vi "XYZ Software.vi"() -> ()   [LabVIEW 2020]
doc: "This was the initial version checking out system parameters and figuring out what each ASCII command does. The other file within this folder is setup to be able to send consecutive commands to the scanning rig controller."
uses:
  <instrlib>/Arcus Ethernet Driver 1.0.0/ArcusEthernetComm/classes/Controller/_Controller.lvclass
panel:
  in  "Program Stop":bool
  in  "Tab Control":T1(tab)
  in  "Scanning Rig Connection":T2
  out "Scanning Rig Disconnection":T2
  out "Current Z Vel (pps)":string
  out "Current Y Vel (pps)":string
  out "Current X Vel (pps)":string
  in  "Set HS Vel (pps)":string
  out "Current Decel (ms^2)":string
  out "Current LS Vel (pps)":string
  out "Current HS Vel (pps)":string
  in  "Set Accel (ms^2)":string
  out "Current Accel (ms^2)":string
  out "Home":bool
  out "Current Z Position":string
  out "Current X Position":string
  out "Current Y Position":string
  in  "Safe Motion Stop":bool
  in  "Direction":string(combo)
  in  "Axis":enum16{"X", "Y", "Z"}(ring)
  in  "Move":bool
  in  "Number of Z Steps":string
  in  "Number of Y Steps":string
  in  "Number of X Steps":string
  out "Z":bool
  out "Y":bool
  out "X":bool
  in  "Home":bool
  in  "Axis":enum16{"X", "Y", "Z"}(ring)
  in  "Direction":string(combo)
  # "`"
  # "GREEN - Operational\nRED - Activate Safe Stop"
  # "HOMING FUNCTION HAS MULTIPLE MODES\nSEE MANUAL"
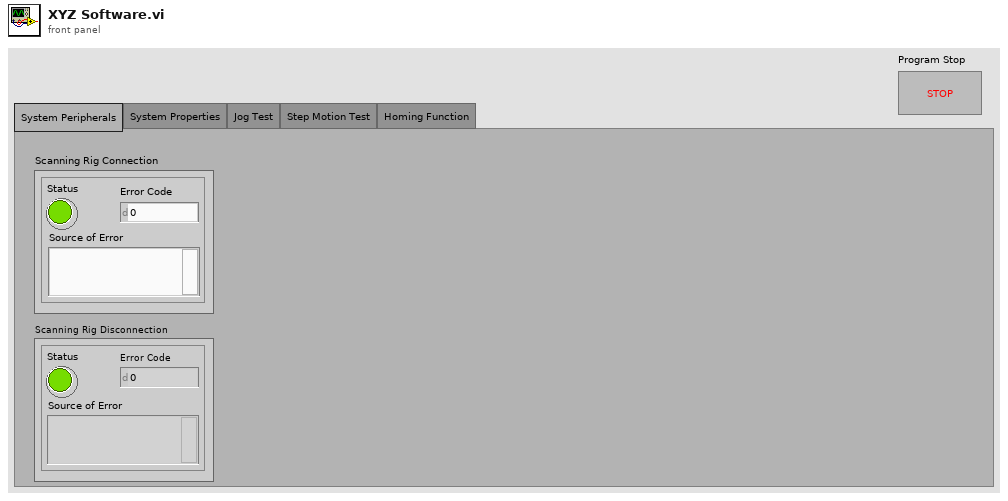
[diagram p1: front panel]
types:
  T1 = enum32{"System Peripherals", "System Properties", "Jog Test", "Step Motion Test", "Homing Function"}
  T2 = cluster{"Status":bool, "Error Code":i32, "Source of Error":string}
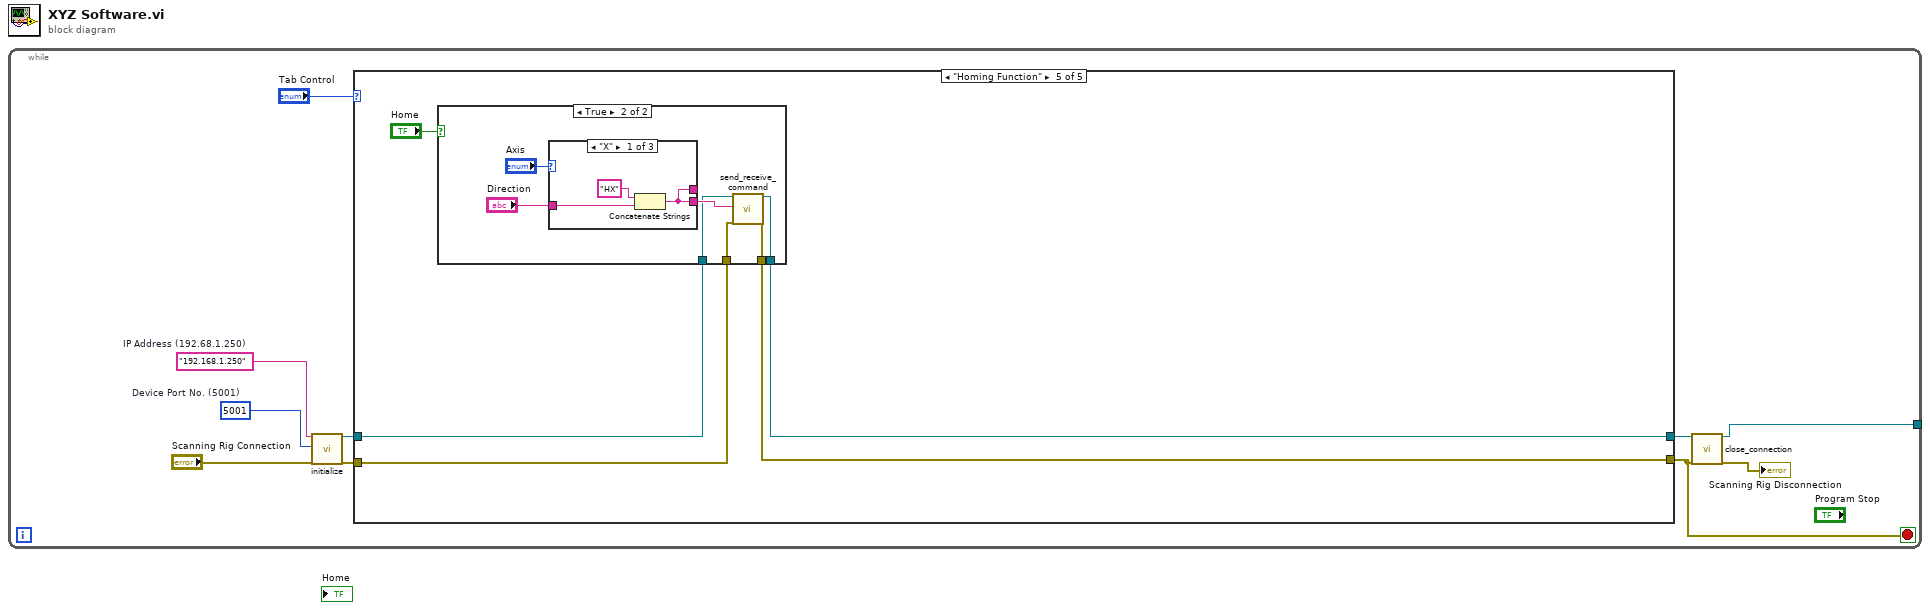
[diagram p0: block diagram]
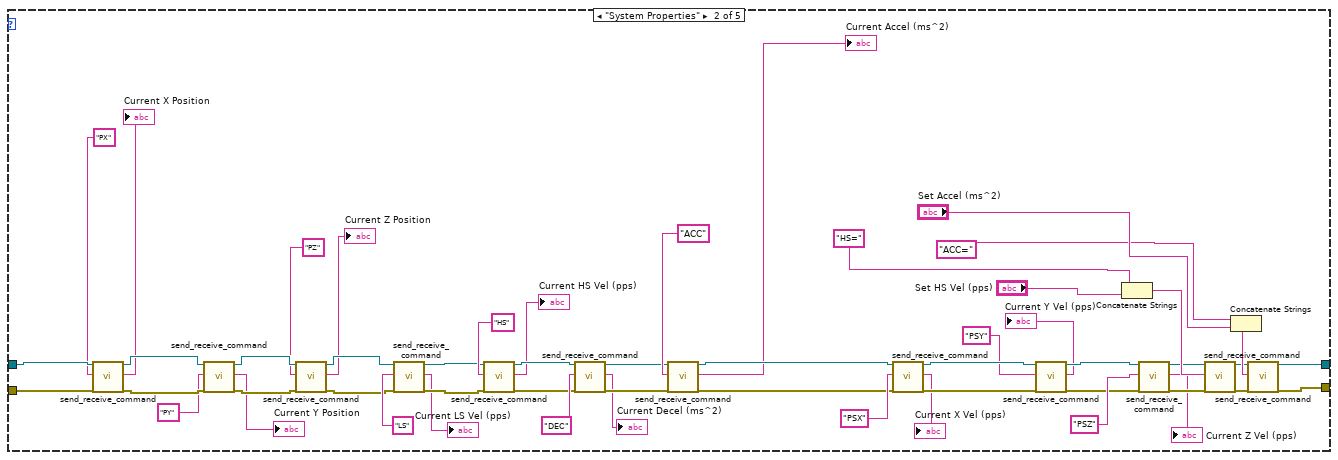
[diagram p3: hidden frame]
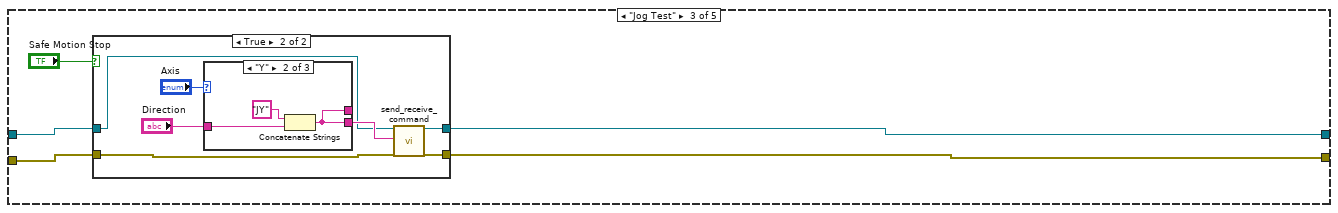
[diagram p4: hidden frame]
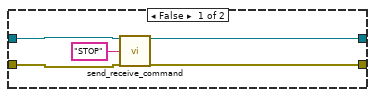
[diagram p5: hidden frame]
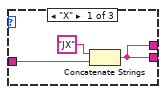
[diagram p6: hidden frame]
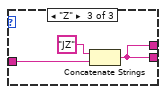
[diagram p7: hidden frame]
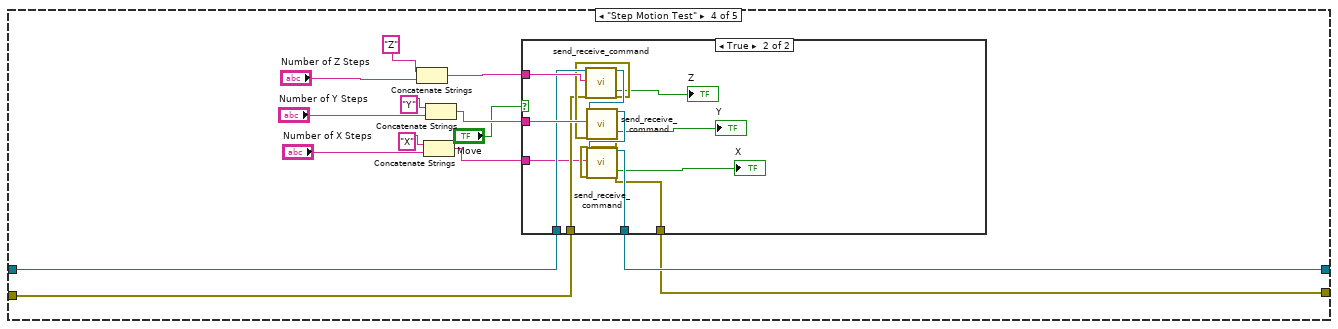
[diagram p8: hidden frame]
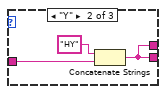
[diagram p11: hidden frame]
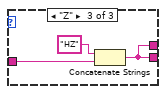
[diagram p12: hidden frame]
diagram:
  n1 = while {
    tunnel: [w4] -> _
    stop <- w1 stop-if-true
    w9 = u16 5001  # Device Port No. (5001)
    w10 = "192.168.1.250"  # IP Address (192.68.1.250)
    n2 = call <instrlib>:"initialize.vi"("ip_address (in)"=w10, "dev_port(def=5001)"=w9, "error in (no error)"="Scanning Rig Connection") -> ("reference (out)"=w6:refnum<class "_Controller.lvclass">, "error out"=w7:errorcluster)  [unwired: 15 in]
    n3 = case shown="\"Homing Function\"" "Tab Control" {
      tunnel: w6 -> [w12 w52 w69 w96 w124]
      tunnel: w7 -> [w11 w43 w68 w93 w121]
      tunnel: [w11 w28 w66 w94 w122] -> w1
      tunnel: [w12 w31 w67 w95 w123] -> w5
      frame "System Peripherals" {
      }
      frame "System Properties" {
        n4 = call <instrlib>:"send_receive_command.vi"("reference (in)"=w52, "ASCII Command (in)"="PX", "error in (no error)"=w43) -> ("reference (out)"=w51:refnum<class "_Controller.lvclass">, "response (out)"=→"Current X Position":string, "error out"=w42:errorcluster)  [unwired: 12 in, 2 out]
        n5 = call <instrlib>:"send_receive_command.vi"("reference (in)"=w51, "ASCII Command (in)"="PY", "error in (no error)"=w42) -> ("reference (out)"=w50:refnum<class "_Controller.lvclass">, "response (out)"=→"Current Y Position":string, "error out"=w41:errorcluster)  [unwired: 12 in, 2 out]
        n6 = call <instrlib>:"send_receive_command.vi"("reference (in)"=w50, "ASCII Command (in)"="PZ", "error in (no error)"=w41) -> ("reference (out)"=w49:refnum<class "_Controller.lvclass">, "response (out)"=→"Current Z Position":string, "error out"=w40:errorcluster)  [unwired: 12 in, 2 out]
        n7 = call <instrlib>:"send_receive_command.vi"("reference (in)"=w49, "ASCII Command (in)"="LS", "error in (no error)"=w40) -> ("reference (out)"=w48:refnum<class "_Controller.lvclass">, "response (out)"=→"Current LS Vel (pps)":string, "error out"=w39:errorcluster)  [unwired: 12 in, 2 out]
        n8 = call <instrlib>:"send_receive_command.vi"("reference (in)"=w48, "ASCII Command (in)"="HS", "error in (no error)"=w39) -> ("reference (out)"=w47:refnum<class "_Controller.lvclass">, "response (out)"=→"Current HS Vel (pps)":string, "error out"=w38:errorcluster)  [unwired: 12 in, 2 out]
        n9 = call <instrlib>:"send_receive_command.vi"("reference (in)"=w47, "ASCII Command (in)"="DEC", "error in (no error)"=w38) -> ("reference (out)"=w18:refnum<class "_Controller.lvclass">, "response (out)"=→"Current Decel (ms^2)":string, "error out"=w37:errorcluster)  [unwired: 12 in, 2 out]
        n10 = call <instrlib>:"send_receive_command.vi"("reference (in)"=w18, "ASCII Command (in)"="ACC", "error in (no error)"=w37) -> ("reference (out)"=w46:refnum<class "_Controller.lvclass">, "response (out)"=→"Current Accel (ms^2)":string, "error out"=w36:errorcluster)  [unwired: 12 in, 2 out]
        n11 = call <instrlib>:"send_receive_command.vi"("reference (in)"=w46, "ASCII Command (in)"="PSX", "error in (no error)"=w36) -> ("reference (out)"=w45:refnum<class "_Controller.lvclass">, "response (out)"=→"Current X Vel (pps)":string, "error out"=w35:errorcluster)  [unwired: 12 in, 2 out]
        n12 = call <instrlib>:"send_receive_command.vi"("reference (in)"=w45, "ASCII Command (in)"="PSY", "error in (no error)"=w35) -> ("reference (out)"=w44:refnum<class "_Controller.lvclass">, "response (out)"=→"Current Y Vel (pps)":string, "error out"=w34:errorcluster)  [unwired: 12 in, 2 out]
        n13 = Concatenate Strings("HS=" ("string"), "Set HS Vel (pps)") -> (w62:string)
        n14 = call <instrlib>:"send_receive_command.vi"("reference (in)"=w44, "ASCII Command (in)"="PSZ", "error in (no error)"=w34) -> ("reference (out)"=w33:refnum<class "_Controller.lvclass">, "response (out)"=→"Current Z Vel (pps)":string, "error out"=w30:errorcluster)  [unwired: 12 in, 2 out]
        n15 = call <instrlib>:"send_receive_command.vi"("reference (in)"=w33, "ASCII Command (in)"=w62, "error in (no error)"=w30) -> ("reference (out)"=w32:refnum<class "_Controller.lvclass">, "error out"=w29:errorcluster)  [unwired: 12 in, 3 out]
        n16 = Concatenate Strings("ACC=" ("string"), "Set Accel (ms^2)") -> (w53:string)
        n17 = call <instrlib>:"send_receive_command.vi"("reference (in)"=w32, "ASCII Command (in)"=w53, "error in (no error)"=w29) -> ("reference (out)"=w31:refnum<class "_Controller.lvclass">, "error out"=w28:errorcluster)  [unwired: 12 in, 3 out]
      }
      frame "Jog Test" {
        n18 = case shown="True" "Safe Motion Stop" {
          tunnel: w69 -> [w73 w79]
          tunnel: w68 -> [w72 w78]
          tunnel: [w70 w77] -> w67
          tunnel: [w71 w76] -> w66
          frame False {
            n19 = call <instrlib>:"send_receive_command.vi"("reference (in)"=w73, "ASCII Command (in)"="STOP", "error in (no error)"=w72) -> ("reference (out)"=w70:refnum<class "_Controller.lvclass">, "error out"=w71:errorcluster)  [unwired: 12 in, 3 out]
          }
          frame True {
            n20 = case shown="\"Y\"" "Axis" {
              tunnel: [w82 w85 w88] -> w81
              tunnel: "Direction" -> [w83 w86 w89]
              tunnel: [w82 w85 w88] -> _
              frame "X" {
                n21 = Concatenate Strings("JX", w83) -> (w82:string)
              }
              frame "Y" {
                n22 = Concatenate Strings("JY", w86) -> (w85:string)
              }
              frame "Z" {
                n23 = Concatenate Strings("JZ", w89) -> (w88:string)
              }
            }
            n24 = call <instrlib>:"send_receive_command.vi"("reference (in)"=w79, "ASCII Command (in)"=w81, "error in (no error)"=w78) -> ("reference (out)"=w77:refnum<class "_Controller.lvclass">, "error out"=w76:errorcluster)  [unwired: 12 in, 3 out]
          }
        }
      }
      frame "Step Motion Test" {
        n25 = Concatenate Strings("Z" ("string"), "Number of Z Steps") -> (w99:string)
        n26 = Concatenate Strings("X" ("string"), "Number of X Steps") -> (w97:string)
        n27 = Concatenate Strings("Y" ("string"), "Number of Y Steps") -> (w98:string)
        n28 = case shown="True" "Move" {
          tunnel: w99 -> [_ w120]
          tunnel: w98 -> [_ w119]
          tunnel: w97 -> [_ w110]
          tunnel: w96 -> [w105 w118]
          tunnel: [w105 w115] -> w95
          tunnel: [w106 w112] -> w94
          tunnel: w93 -> [w106 w111]
          frame False {
          }
          frame True {
            n29 = call <instrlib>:"send_receive_command.vi"("reference (in)"=w118, "ASCII Command (in)"=w120, "error in (no error)"=w111) -> ("reference (out)"=w117:refnum<class "_Controller.lvclass">, "success?"=→"Z":bool, "error out"=w114:errorcluster)  [unwired: 12 in, 2 out]
            n30 = call <instrlib>:"send_receive_command.vi"("reference (in)"=w117, "ASCII Command (in)"=w119, "error in (no error)"=w114) -> ("reference (out)"=w116:refnum<class "_Controller.lvclass">, "success?"=→"Y":bool, "error out"=w113:errorcluster)  [unwired: 12 in, 2 out]
            n31 = call <instrlib>:"send_receive_command.vi"("reference (in)"=w116, "ASCII Command (in)"=w110, "error in (no error)"=w113) -> ("reference (out)"=w115:refnum<class "_Controller.lvclass">, "success?"=→"X":bool, "error out"=w112:errorcluster)  [unwired: 12 in, 2 out]
          }
        }
      }
      frame "Homing Function" {
        n32 = case shown="True" "Home" {
          tunnel: w124 -> [w126 w131]
          tunnel: [w126 w130] -> w123
          tunnel: [w127 w129] -> w122
          tunnel: w121 -> [w127 w128]
          frame False {
          }
          frame True {
            n33 = case shown="\"X\"" "Axis" {
              tunnel: [w135 w138 w141] -> w132
              tunnel: "Direction" -> [w136 w139 w142]
              tunnel: [w135 w138 w141] -> _
              frame "X" {
                n34 = Concatenate Strings("HX", w136) -> (w135:string)
              }
              frame "Y" {
                n35 = Concatenate Strings("HY", w139) -> (w138:string)
              }
              frame "Z" {
                n36 = Concatenate Strings("HZ", w142) -> (w141:string)
              }
            }
            n37 = call <instrlib>:"send_receive_command.vi"("reference (in)"=w131, "ASCII Command (in)"=w132, "error in (no error)"=w128) -> ("reference (out)"=w130:refnum<class "_Controller.lvclass">, "error out"=w129:errorcluster)  [unwired: 12 in, 3 out]
          }
        }
      }
    }
    n38 = call <instrlib>:"close_connection.vi"("reference (in)"=w5, "error in (no error)"=w1) -> ("reference (out)"=w4:refnum<class "_Controller.lvclass">, "error out"=→"Scanning Rig Disconnection":errorcluster)  [unwired: 16 in]
  }
